vi "TempSubVI.vi"() -> (3 "temp":dbl)   [LabVIEW 2019]
doc: "Genera una temperatura aleatòria entre -40 i 80º."
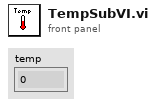
[diagram p1: front panel]
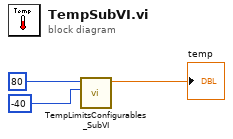
[diagram p0: block diagram]
diagram:
  n1 = call "TempLimitsConfigurables_SubVI.vi"("TempMin"=-40, "TempMax"=80) -> ("RandomTemp"=→"temp":dbl)  [unwired: 9 in]
